vi "SetState.vi"(0 "object in":refnum<class "TrafficLight.lvclass">, 2 "State":refnum<class "State.lvclass">, 5 "Error In":errorcluster) -> (14 "object out":refnum<class "TrafficLight.lvclass">, 19 "Error Out":errorcluster)   [LabVIEW 2024, in "TrafficLight.lvclass"]
uses:
  TrafficLight.lvclass
  TrafficLight.lvclass/TrafficLight.ctl
  State_interface/State.lvclass
panel:
  # "Connector Pane"
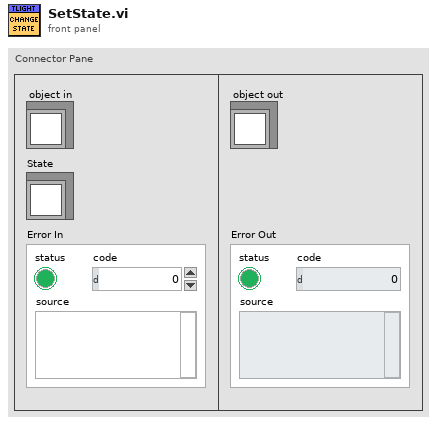
[diagram p1: front panel]
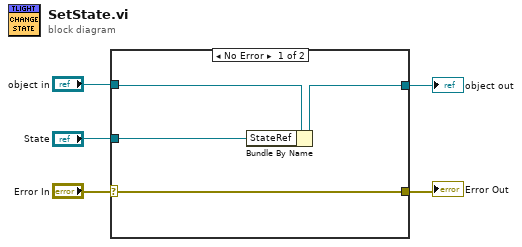
[diagram p0: block diagram]
diagram:
  n1 = case shown="No Error" "Error In" {
    selector: "Error In" -> [w9 w11]
    tunnel: [w9 w11] -> w4
    tunnel: [w7 w10] -> w2
    tunnel: "object in" -> [w8 w10]
    tunnel: "State" -> [w6 _]
    frame No Error {
      n2 = Bundle By Name(cluster=w8, "StateRef"=w6) -> (w7:refnum<class "TrafficLight.lvclass">)
    }
    frame Error {
    }
  }
  "Error Out" <- w4
  "object out" <- w2
